vi "2039_hw UpdateMecanumMotors.vi"(5 "VComp Scaling":bool, 6 "Rear Right":dbl, 7 "Rear Left":dbl, 8 "error in":errorcluster, 9 "Front Right":dbl, 10 "Front Left":dbl, 11 "RobotDriveDevRef in":T1) -> (0 "error out":errorcluster, 2 "Motor Values":dbl[](array[numeric]), 3 "RobotDriveDevRef out":T1)   [LabVIEW 2016, in "2039lib.lvlib"]
uses:
  2039lib.lvlib
  <vilib>/Rock Robotics/WPI/RobotDrive/WPI_RobotDriveDevRef.ctl
  <vilib>/Rock Robotics/WPI/MotorControl/WPI_MotorControlDeviceRef.ctl
  <vilib>/Rock Robotics/WPI/MotorControl/WPI_MotorControlType.ctl
  <vilib>/Rock Robotics/SystemInterfaces/DIO/FPGA_DIOPWMChannel.ctl
  <vilib>/Rock Robotics/WPI/PWM/WPI_PWMDeadband.ctl
  <vilib>/Rock Robotics/WPI/RobotDrive/WPI_RobotDriveMotorSelectorEnum.ctl
  <vilib>/Rock Robotics/WPI/RobotDrive/WPI_RobotDriveSafetyCheck.vi
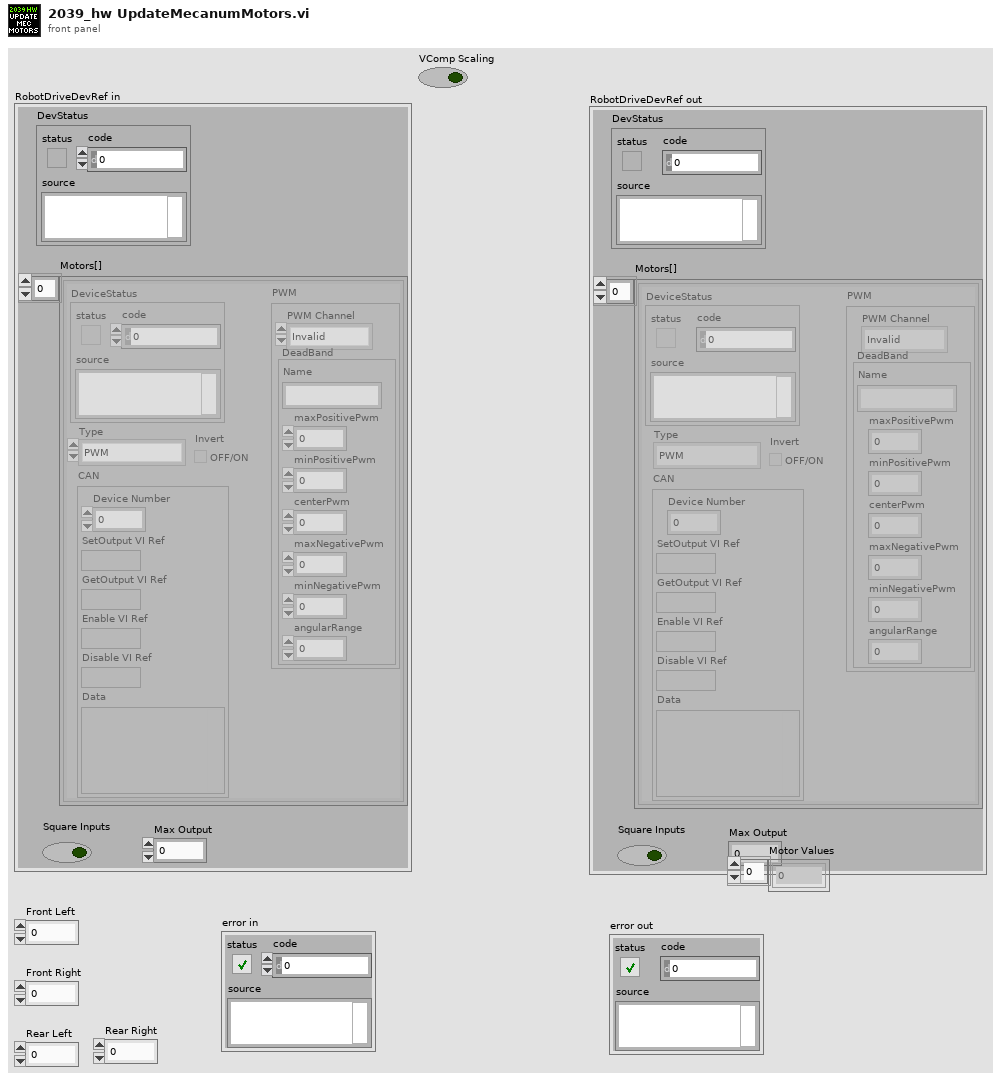
[diagram p1: front panel]
types:
  T1 = typedef "WPI_RobotDriveDevRef.ctl" = cluster{"DevStatus":errorcluster, "Motors[]":T2[], "Square Inputs":bool, "Max Output":dbl}
  T2 = typedef "WPI_MotorControlDeviceRef.ctl" = cluster{"DeviceStatus":errorcluster, "Type":T3, "PWM":cluster{"PWM Channel":T4, "DeadBand":T5}, "CAN":cluster{"Device Number":u8, "SetOutput VI Ref":variant, "GetOutput VI Ref":variant, "Enable VI Ref":variant, "Disable VI Ref":variant, "Data":variant}, "Invert":bool}
  T3 = typedef "WPI_MotorControlType.ctl" = enum16{"PWM", "CAN"}
  T4 = typedef "FPGA_DIOPWMChannel.ctl" = enum8{"PWM 0", "PWM 1", "PWM 2", "PWM 3", "PWM 4", "PWM 5", "PWM 6", "PWM 7", "PWM 8", "PWM 9", "PWM MXP 0", "PWM MXP 1", "PWM MXP 2", "PWM MXP 3", "PWM MXP 4", "PWM MXP 5", "PWM MXP 6", "PWM MXP 7", "PWM MXP 8", "PWM MXP 9", "Invalid"}
  T5 = typedef "WPI_PWMDeadband.ctl" = cluster{"Name":string, "maxPositivePwm":i32, "minPositivePwm":i32, "centerPwm":i32, "maxNegativePwm":i32, "minNegativePwm":i32, "angularRange":u16}
  T6 = typedef "WPI_RobotDriveMotorSelectorEnum.ctl" = enum16{"Rear Left Motor", "Rear Right Motor", "Front Left Motor", "Front Right Motor"}
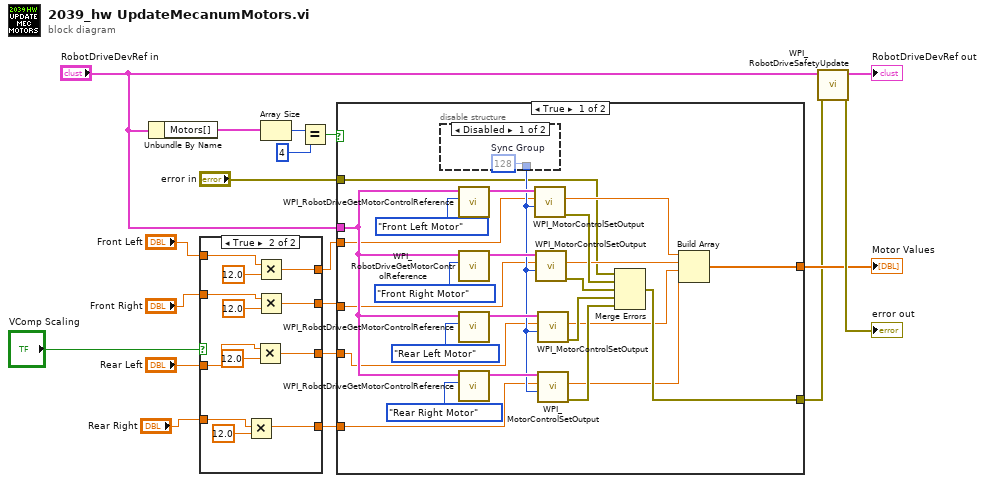
[diagram p0: block diagram]
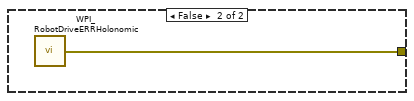
[diagram p4: hidden frame]
diagram:
  n1 = Unbundle By Name("RobotDriveDevRef in") -> ("Motors[]"=w15:T2[])
  n2 = case shown="True" "VComp Scaling" {
    tunnel: "Front Left" -> [w23 w34]
    tunnel: [w23 w33] -> w8
    tunnel: "Front Right" -> [w22 w29]
    tunnel: "Rear Left" -> [w21 w28]
    tunnel: "Rear Right" -> [w20 w27]
    tunnel: [w22 w26] -> w4
    tunnel: [w21 w25] -> w3
    tunnel: [w20 w24] -> w2
    frame False {
    }
    frame True {
      n3 = Multiply(x=w27, y=12.0) -> (x*y=w24:dbl)
      n4 = Multiply(x=w28, y=12.0) -> (x*y=w25:dbl)
      n5 = Multiply(x=w34, y=12.0) -> (x*y=w33:dbl)
      n6 = Multiply(x=w29, y=12.0) -> (x*y=w26:dbl)
    }
  }
  n7 = Array Size(array=w15) -> (size(s)=w11:i32)
  n8 = Equal?(x=w11, y=4) -> (x = y?=w13:bool)
  n9 = case shown="True" w13 {
    tunnel: w8 -> [w38 _]
    tunnel: w4 -> [w39 _]
    tunnel: "RobotDriveDevRef in" -> [w52 _]
    tunnel: [w47 w62] -> w14
    tunnel: w2 -> [w40 _]
    tunnel: [w41 _] -> w16
    tunnel: "error in" -> [w37 _]
    tunnel: w3 -> [w36 _]
    frame True {
      n10 = disable-structure shown="Disabled" {
        disable-tunnel: [w61 _] -> w46
        frame Disabled {
          w61 = u8 128  # Sync Group
        }
        frame Enabled {
        }
      }
      n11 = call <vilib>:"WPI_RobotDriveGetMotorControlReference.vi"("MotorIndex"=WPI_RobotDriveMotorSelectorEnum."Front Left Motor", "RobotDriveDevRef"=w52) -> ("MotorControlDeviceRef"=w60:T2)  [unwired: 9 out]
      n12 = call <vilib>:"WPI_RobotDriveGetMotorControlReference.vi"("MotorIndex"=WPI_RobotDriveMotorSelectorEnum."Front Right Motor", "RobotDriveDevRef"=w52) -> ("MotorControlDeviceRef"=w58:T2)  [unwired: 9 out]
      n13 = call <vilib>:"WPI_RobotDriveGetMotorControlReference.vi"("MotorIndex"=WPI_RobotDriveMotorSelectorEnum."Rear Left Motor", "RobotDriveDevRef"=w52) -> ("MotorControlDeviceRef"=w59:T2)  [unwired: 9 out]
      n14 = call <vilib>:"WPI_RobotDriveGetMotorControlReference.vi"("MotorIndex"=WPI_RobotDriveMotorSelectorEnum."Rear Right Motor", "RobotDriveDevRef"=w52) -> ("MotorControlDeviceRef"=w57:T2)  [unwired: 9 out]
      n15 = call <vilib>:"WPI_MotorControlSetOutput.vi"("options"=w46, "Output"=w38, "MotorControlDevRef"=w60) -> ("error out"=w48:errorcluster, "Motor Output"=w45:dbl)  [unwired: 1 in, 6 out]
      n16 = call <vilib>:"WPI_MotorControlSetOutput.vi"("options"=w46, "Output"=w39, "MotorControlDevRef"=w58) -> ("error out"=w49:errorcluster, "Motor Output"=w44:dbl)  [unwired: 1 in, 6 out]
      n17 = call <vilib>:"WPI_MotorControlSetOutput.vi"("options"=w46, "Output"=w36, "MotorControlDevRef"=w59) -> ("error out"=w50:errorcluster, "Motor Output"=w43:dbl)  [unwired: 1 in, 6 out]
      n18 = call <vilib>:"WPI_MotorControlSetOutput.vi"("options"=w46, "Output"=w40, "MotorControlDevRef"=w57) -> ("error out"=w51:errorcluster, "Motor Output"=w42:dbl)  [unwired: 1 in, 6 out]
      n19 = Merge Errors(w37, w48, w49, w50, w51) -> (w47:errorcluster)
      n20 = Build Array(w45, w44, w43, w42) -> (w41:dbl[])
    }
    frame False {
      n21 = call <vilib>:"WPI_RobotDriveERRHolonomic.vi"() -> ("error out"=w62:errorcluster)
    }
  }
  "Motor Values" <- w16
  n22 = call <vilib>:"WPI_RobotDriveSafetyUpdate.vi"("error in (no error)"=w14, "RobotDriveDevRef"="RobotDriveDevRef in") -> ("error out"=→"error out":errorcluster, "RobotDriveDevRef"=→"RobotDriveDevRef out":T1)  [unwired: 8 out]
